vi "setUp.vi"(8 "error in (no error)":errorcluster, 11 "reference in":refnum<class "Time Filter Tester.lvclass">) -> (0 "error out":errorcluster, 3 "reference out":refnum<class "Time Filter Tester.lvclass">)   [LabVIEW 2016, in "Time Filter Tester.lvclass"]
doc: "setUp runs prior to the test method during test execution. Use this method to initialize any object data required by your tests."
uses:
  Time Filter Tester.lvclass
  C:/Program Files (x86)/National Instruments/LabVIEW 2016/vi.lib/addons/_JKI Toolkits/VI Tester/TestCase.llb/TestCase.lvclass
  Core/Assert API Components/Filter Configurations/Time Filters/Time Filters.lvclass
  Time Filter Tester.lvclass/Time Filter Tester.ctl
  <vilib>/addons/_JKI Toolkits/VI Tester/TestCase.llb/TestCase.lvclass
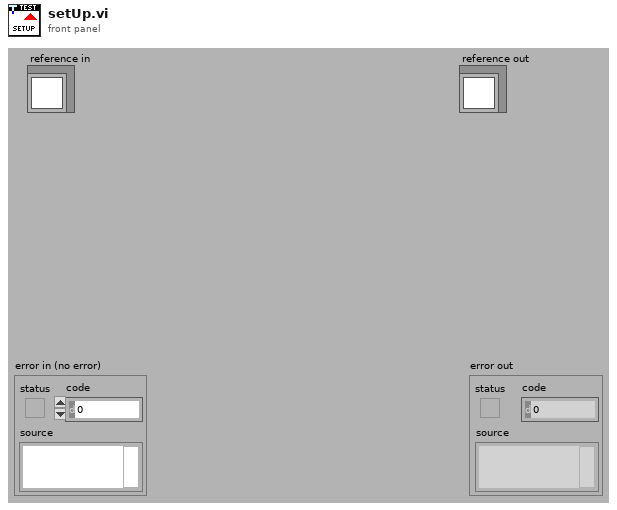
[diagram p1: front panel]
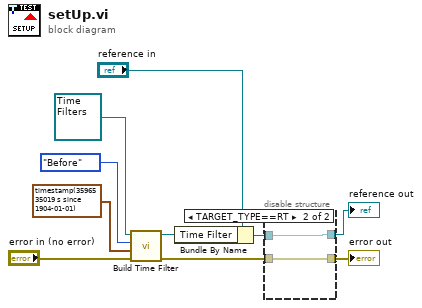
[diagram p0: block diagram]
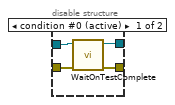
[diagram p2: hidden frame]
diagram:
  n1 = call "Build Time Filter.vi"("error in (no error)"="error in (no error)", "Comparison Timestamp"=timestamp(3596535019.229245 s since 1904-01-01), "Comparison Method"=enum16{"Before", "After"}."Before", "Time Filters in"=refnum<class "Time Filters.lvclass"> refnum) -> ("error out"=w1:errorcluster, "Time Filters out"=w2:refnum<class "Time Filters.lvclass">)  [unwired: 6 in]
  n2 = Bundle By Name(cluster="reference in", "Time Filter"=w2) -> (w7:refnum<class "Time Filter Tester.lvclass">)
  n3 = disable-structure shown="TARGET_TYPE==RT" {
    disable-tunnel: w1 -> [w14 w15]
    disable-tunnel: [w13 w15] -> w10
    disable-tunnel: [w12 w16] -> w8
    disable-tunnel: w7 -> [w11 w16]
    frame condition #0 (active) {
      n4 = call <vilib>:"WaitOnTestComplete.vi"("error in (no error)"=w14, "TestCase in"=w11) -> ("error out"=w13:errorcluster, "TestCase out"=w12:refnum<class "Time Filter Tester.lvclass">)  [unwired: 8 in]
    }
    frame condition #1 {
    }
  }
  "error out" <- w10
  "reference out" <- w8
